vi "GET_2D_Array_Interpolated_to_size_of_image.vi"(6 "Truncate negative values (F)":bool=TRUE, 7 "Method":i32(ring) items=["nearest", "bilinear", "bicubic", "bicubic spline"], 8 "# bins per axis":i32=64, 9 "Y image size":i32=480, 10 "X image size":i32=480, 11 "Array or pixmap in":u32[][](array[numeric])) -> (2 "Interp. size":i32[](array[numeric]), 3 "Array or pixmap out":dbl[][](array[numeric]))   [LabVIEW 2018, in "Tracker.lvlib"]
uses:
  <vilib>/gmath/interp.llb/Create Mesh Grid (2D) (x,y arrays).vi
  <vilib>/gmath/interp.llb/Interpolate 2D (2d X,Y).vi
  Tracker.lvlib
  <vilib>/gmath/NI_Gmath.lvlib
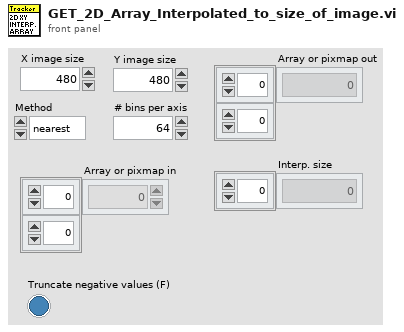
[diagram p1: front panel]
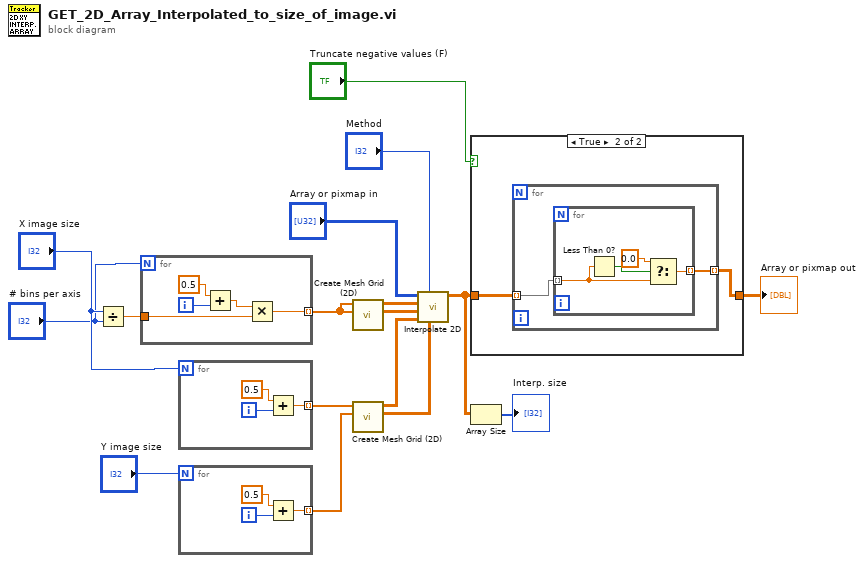
[diagram p0: block diagram]
diagram:
  n1 = Divide(x="X image size", y="# bins per axis") -> (x/y=w13:dbl)
  n2 = for {
    N: "# bins per axis" -> [_]
    tunnel: [w21] -> w6 mode=indexing
    tunnel: w13 -> [w20]
    i -> [w22]
    n3 = Add(x=0.5, y=w22) -> (x+y=w19:dbl)
    n4 = Multiply(x=w19, y=w20) -> (x*y=w21:dbl)
  }
  n5 = for {
    N: "X image size" -> [_]
    tunnel: [w24] -> w14 mode=indexing
    i -> [w25]
    n6 = Add(x=0.5, y=w25) -> (x+y=w24:dbl)
  }
  n7 = for {
    N: "Y image size" -> [_]
    tunnel: [w27] -> w4 mode=indexing
    i -> [w28]
    n8 = Add(x=0.5, y=w28) -> (x+y=w27:dbl)
  }
  n9 = call-poly <vilib>:"Create Mesh Grid (2D).vi"("y domain"=w6, "x domain"=w6) -> ("Y"=w9:dbl[][], "X"=w8:dbl[][])  [unwired: 7 in, 1 out]
  n10 = call-poly <vilib>:"Create Mesh Grid (2D).vi"("y domain"=w4, "x domain"=w14) -> ("Y"=w16:dbl[][], "X"=w15:dbl[][])  [unwired: 7 in, 1 out]
  n11 = call-poly <vilib>:"Interpolate 2D.vi"("yi"=w16, "method"="Method", "xi"=w15, "Y"=w9, "X"=w8, "Z"="Array or pixmap in") -> ("zi"=w2:dbl[][])  [unwired: 2 in, 3 out]
  n12 = case shown="True" "Truncate negative values (F)" {
    tunnel: w2 -> [w29 w31]
    tunnel: [w29 w30] -> w1
    frame False {
    }
    frame True {
      n13 = for {
        tunnel: w31 -> [w32] mode=indexing
        tunnel: [w33] -> w30 mode=indexing
        n14 = for {
          tunnel: [w37] -> w33 mode=indexing
          tunnel: w32 -> [w35] mode=indexing
          n15 = Less Than 0?(x=w35) -> (x < 0?=w36:bool)
          n16 = Select(t=0.0, s=w36, f=w35) -> (s? t:f=w37:dbl)
        }
      }
    }
  }
  "Array or pixmap out" <- w1
  n17 = Array Size(array=w2) -> (size(s)=→"Interp. size":i32[])
